vi "Broadcast to uServices in locale.vi"(0 "Guardian in":refnum<class "Guardian.lvclass">, 5 "Event type":T1=enum."Message", 7 "Message":string, 9 "Data":variant, 11 "error in (no error)":errorcluster) -> (4 "Guardian out":refnum<class "Guardian.lvclass">, 15 "error out":errorcluster)   [LabVIEW 2026, in "TALOS.lvlib" / "Guardian.lvlib" / "Guardian.lvclass"]
uses:
  Guardian.lvclass
  Father of all uServices/Father of all uServices/Event Handler Items.ctl
  Classes/uService List/uService List.lvclass/uService List.ctl
  Father of all uServices/Father of all uServices Messages/Event Handler Msg/Event Handler Msg.lvclass/Event Handler Msg.ctl
  Ancestor/Ancestor/Ancestor.lvclass/Ancestor.ctl
  Classes/uService List/Get all Queue.vi
  Support VIs/Generate Error.vi
  FGV/Error Memory/Get Error Description.vi
  Support VIs/Get PC name.vi
  Ancestor/Ancestor/Read ID.vi
  Support VIs/Get Class Name.vi
  <vilib>/Utility/error.llb/Clear Errors.vi
  FGV/Error Memory/Error Memory Core.vi
  <vilib>/AdvancedString/Delimited String to 1D String Array.vi
  <vilib>/AdvancedString/Delimited String to 1D String Array (string).vi
  Support VIs/Circus Root Path.vi
  FGV/Error Memory/Error Crt Lvl checker.vi
  FGV/Error Memory/Error Memory Core.vi/40c8088d-b597-4017-91af-faa98e00292e.vi
  FGV/Error Memory/Error Memory Core.vi/d4a3ab98-063c-4e44-b43d-fbdcfe6c2be2.vi
  builds/Actor Framework PPL/Actor Framework.lvlibp/1abvi3w/vi.lib/ActorFramework/Message Enqueuer/Enqueue.vi
  Support VIs/Global Memory.vi
  <vilib>/Utility/LVClass/Get LV Class Name.vi
  Support VIs/Is in Packed Library.vi
  Support VIs/TALOS Root path.vi
  Support VIs/Read CSV worksheet.vi
  Support VIs/Global Constants.vi
  <vilib>/Utility/error.llb/General Error Handler.vi
  Support VIs/Error Log.vi
  Father of all uServices/Father of all uServices Messages/Event Handler Msg/Event Handler Msg.lvclass
  Ancestor/Ancestor/Ancestor.lvclass
  <vilib>/Comparison/Equal/Equal Functor/Equal Functor.lvclass
  Classes/uService List/uService List.lvclass
  TALOS.lvlib
  Father of all uServices/Father of all uServices/Father of all uServices.lvclass
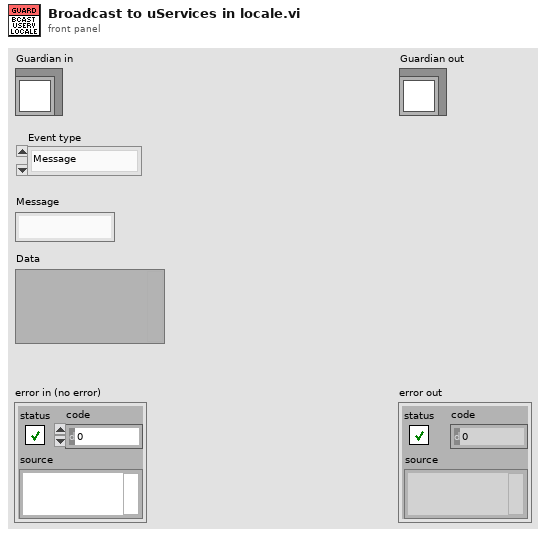
[diagram p1: front panel]
types:
  T1 = typedef "TALOS.lvlib/Father of all uServices.lvlib/Father of all uServices.lvclass/Event Handler Items.ctl" = enum16{"Button Pressed", "Message", "Ready to launch?", "Safe Mode", "Start RUN", "Stop RUN"}
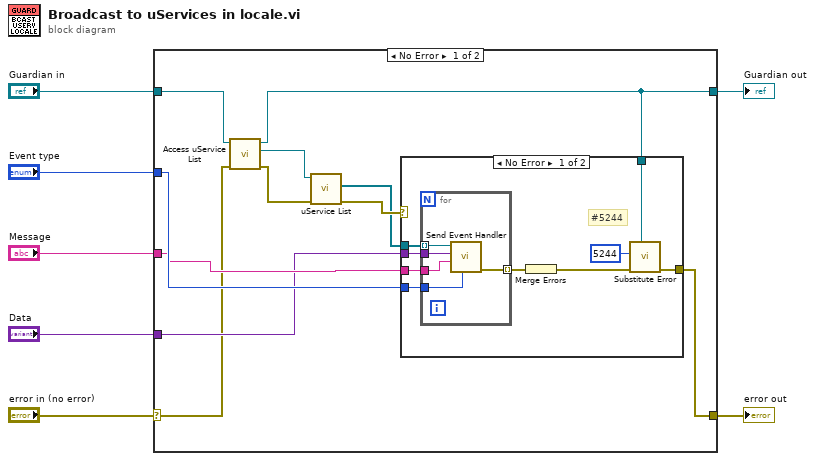
[diagram p0: block diagram]
diagram:
  n1 = case shown="No Error" "error in (no error)" {
    selector: "error in (no error)" -> [w12 w35]
    tunnel: [w14 w35] -> w7
    tunnel: "Guardian in" -> [w13 w34]
    tunnel: [w8 w34] -> w4
    tunnel: "Event type" -> [w18 _]
    tunnel: "Message" -> [w17 _]
    tunnel: "Data" -> [w16 _]
    frame No Error {
      n2 = call-dynamic "Access uService List.vi"("error in (no error)"=w12, "Ancestor in"=w13) -> ("error out"=w11:errorcluster, "uService List out"=w10:refnum<class "uService List.lvclass">, "Ancestor out"=w8:refnum<class "Guardian.lvclass">)  [unwired: 7 in]
      n3 = call-poly "uService List.vi"("error in (no error)"=w11, "uService List"=w10) -> ("error out"=w15:errorcluster, "All queues"=w9:refnum<class "Message Enqueuer.lvclass">[])  [unwired: 7 in, 1 out]
      n4 = case shown="No Error" w15 {
        selector: w15 -> [_ w33]
        tunnel: w9 -> [w27 _]
        tunnel: w18 -> [w26 _]
        tunnel: w17 -> [w25 _]
        tunnel: w16 -> [w24 _]
        tunnel: [w21 w33] -> w14
        tunnel: w8 -> [w20 _]
        frame No Error {
          # "#5244"
          n5 = for {
            tunnel: w27 -> [w32] mode=indexing
            tunnel: w24 -> [w31]
            tunnel: w25 -> [w30]
            tunnel: w26 -> [w29]
            tunnel: [w28] -> w23 mode=indexing
            n6 = call "Send Event Handler.vi"("Event type"=w29, "Item Name"=w30, "Data"=w31, "Message Enqueuer"=w32) -> ("error out"=w28:errorcluster)  [unwired: 6 in, 1 out]
          }
          n7 = Merge Errors(w23) -> (w22:errorcluster)
          n8 = call "Substitute Error.vi"("LabVIEW Object"=w20, "error in (no error)"=w22, "Error Code"=5244) -> ("error out"=w21:errorcluster)  [unwired: 8 in]
        }
        frame Error {
        }
      }
    }
    frame Error {
    }
  }
  "error out" <- w7
  "Guardian out" <- w4
